vi "PDP Data Collection VI.vi"   [LabVIEW 2014]
uses:
  Robot Global Data.vi
types:
  T1 = enum16{"open", "replace", "create", "open or create", "replace or create", "replace or create with confirmation"}
  T2 = typedef "WPI_DriverStationRobotMode2.ctl" = enum16{"Autonomous Disabled", "Autonomous Enabled", "Teleop Disabled", "Teleop Enabled", "Disconnected", "Finish", "Test Disabled", "Test Enabled", "Emergency Stopped"}
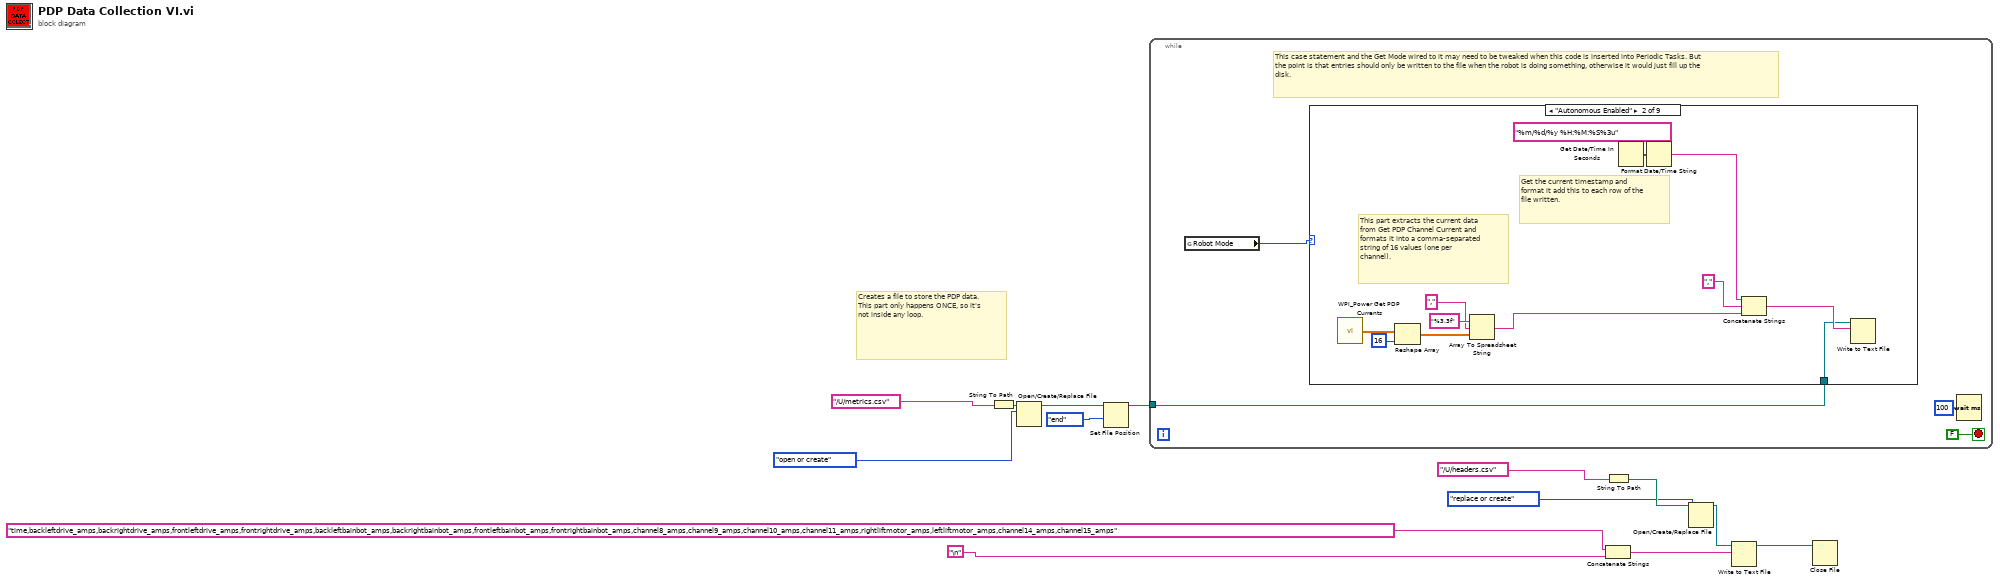
[diagram p0: block diagram]
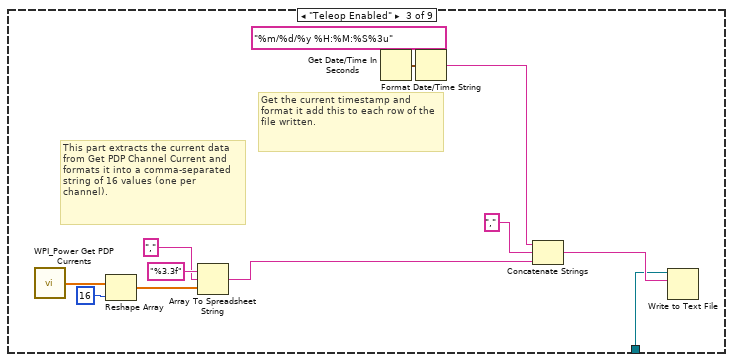
[diagram p3: hidden frame]
diagram:
  # "Creates a file to store the PDP data. This part only happens ONCE, so it's not inside any loop."
  n1 = String To Path(string="/U/metrics.csv") -> (path=w11:path)
  n2 = Open/Create/Replace File(file path (use dialog)=w11, operation (0:open)=T1."open or create") -> (refnum out=w1:refnum<file>)  [unwired: 4 in, 2 out]
  n3 = Set File Position(refnum=w1, from (0:start)=enum16{"start", "end", "current"}."end") -> ()  [unwired: 2 in, 2 out]
  n4 = while {
    tunnel: w1 -> [w14]
    stop <- FALSE stop-if-true
    # "This case statement and the Get Mode wired to it may need to be tweaked when this code is inserted into Periodic Tasks. But the point is that entries should only be written to the file when the robot is doing something, otherwise it would just fill up the disk."
    n5 = global read "Robot Global Data.vi" "Robot Mode"() -> (w15:T2)
    n6 = case shown="\"Autonomous Enabled\"" w15 {
      tunnel: w14 -> [_ w18 w30 _ _ _ _ _ _]
      frame "Autonomous Disabled", Default {
      }
      frame "Autonomous Enabled" {
        # "Get the current timestamp and format it add this to each row of the file written."
        # "This part extracts the current data from Get PDP Channel Current and formats it into a comma-separated string of 16 values (one per channel)."
        n7 = call <vilib>:"WPI_Power Get PDP Currents.vi"() -> ("all currents (A)"=w25:dbl[])  [unwired: 13 in, 2 out]
        n8 = Reshape Array(w25, 16) -> (w29:dbl[])
        n9 = Array To Spreadsheet String(delimiter (Tab)=",", array=w29, 3:"%3.3f" ("format string")) -> (spreadsheet string=w20:string)
        n10 = Get Date/Time In Seconds() -> (seconds since 1Jan1904=w24:timestamp)
        n11 = Format Date/Time String(time format string (%c)="%m/%d/%y %H:%M:%S%3u", seconds (now)=w24) -> (date/time string=w22:string)  [unwired: 1 in]
        n12 = Concatenate Strings(w22, "," ("string"), w20) -> (w19:string)
        n13 = Write to Text File(file (use dialog)=w18, text=w19) -> ()  [unwired: 2 in, 3 out]
      }
      frame "Teleop Enabled" {
        # "Get the current timestamp and format it add this to each row of the file written."
        # "This part extracts the current data from Get PDP Channel Current and formats it into a comma-separated string of 16 values (one per channel)."
        n14 = call <vilib>:"WPI_Power Get PDP Currents.vi"() -> ("all currents (A)"=w37:dbl[])  [unwired: 13 in, 2 out]
        n15 = Reshape Array(w37, 16) -> (w41:dbl[])
        n16 = Array To Spreadsheet String(delimiter (Tab)=",", array=w41, 3:"%3.3f" ("format string")) -> (spreadsheet string=w32:string)
        n17 = Get Date/Time In Seconds() -> (seconds since 1Jan1904=w36:timestamp)
        n18 = Format Date/Time String(time format string (%c)="%m/%d/%y %H:%M:%S%3u", seconds (now)=w36) -> (date/time string=w34:string)  [unwired: 1 in]
        n19 = Concatenate Strings(w34, "," ("string"), w32) -> (w31:string)
        n20 = Write to Text File(file (use dialog)=w30, text=w31) -> ()  [unwired: 2 in, 3 out]
      }
      frame "Disconnected" {
      }
      frame "Finish" {
      }
      frame "Test Disabled" {
      }
      frame "Test Enabled" {
      }
      frame "Emergency Stopped" {
      }
      frame "Teleop Disabled" {
      }
    }
    n21 = Wait (ms)(milliseconds to wait=u32 100) -> ()  [unwired: 1 out]
  }
  n22 = Concatenate Strings("time,backleftdrive_amps,backrightdrive_amps,frontleftdrive_amps,frontrightdrive_amps,backleftbainbot_amps,backrightbainbot_amps,frontleftbainbot_amps,frontrightbainbot_amps,channel8_amps,channel9_amps,channel10_amps,channel11_amps,rightliftmotor_amps,leftliftmotor_amps,channel14_amps,channel15_amps", "\n") -> (w7:string)
  n23 = String To Path(string="/U/headers.csv") -> (path=w5:path)
  n24 = Open/Create/Replace File(file path (use dialog)=w5, operation (0:open)=T1."replace or create") -> (refnum out=w10:refnum<file>)  [unwired: 4 in, 2 out]
  n25 = Write to Text File(file (use dialog)=w10, text=w7) -> (refnum out=w3:refnum<file>)  [unwired: 2 in, 2 out]
  n26 = Close File(refnum=w3) -> ()  [unwired: 1 in, 2 out]
